vi "Broadcast Topics (Global).vi"() -> ()   [LabVIEW 2018]
panel:
  in  "Broadcast Gen":bool=TRUE
  in  "Broadcast ES2":bool=TRUE
  in  "Broadcast ES1":bool=TRUE
  in  "Broadcast PV":bool=TRUE
  in  "Broadcast PCC":bool=TRUE
  in  "Broadcast Load":bool=TRUE
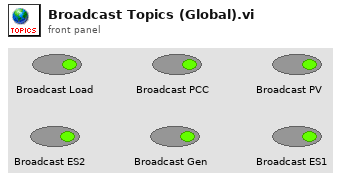
[diagram p1: front panel]
diagram:
